vi "Lab Panel V4.83.vi"() -> ()   [LabVIEW 2013] (continued)
                            n2032 = Bundle By Name("Y"=w3252, "t0"=w3245) -> (w3244:waveform(dbl))  [unwired: 1 in]
                            n2033 = Bundle By Name("Y"=w3251, "t0"=w3245) -> (w3243:waveform(dbl))  [unwired: 1 in]
                            n2034 = Bundle By Name("Y"=w3250, "t0"=w3245) -> (w3242:waveform(dbl))  [unwired: 1 in]
                            n2035 = Bundle By Name("Y"=w3249, "t0"=w3245) -> (w3241:waveform(dbl))  [unwired: 1 in]
                            n2036 = Bundle By Name("Y"=w3248, "t0"=w3245) -> (w3240:waveform(dbl))  [unwired: 1 in]
                            n2037 = Bundle By Name("Y"=w3247, "t0"=w3245) -> (w3239:waveform(dbl))  [unwired: 1 in]
                            n2038 = Bundle By Name("Y"=w3246, "t0"=w3245) -> (w3238:waveform(dbl))  [unwired: 1 in]
                            n2039 = Build Array(w3244, w3243, w3242, w3241, w3240, w3239, w3238) -> (w3237:waveform(dbl)[])
                            n2040 = TDMS Write(0:w3258, 5:"TEST VALUES", 7:w3229, 9:w3237) -> (4:w3228:refnum<k34>, 6:w3227:string, 15:w3226:errorcluster)  [unwired: 2 in, 1 out]
                            n2041 = TDMS Write(0:w3228, 5:w3227, 7:"TIME", 9:w3224, 11:w3226) -> (15:w3223:errorcluster)  [unwired: 1 in, 3 out]
                            n2042 = local write "data file error"(w3223) -> ()
                          }
                        }
                      }
                    }
                  }
                }
              }
              frame #4 {
                n2043 = case shown="True" w3262 {
                  tunnel: w3266 -> [_ w3271]
                  tunnel: w3265 -> [_ w3270]
                  tunnel: w3264 -> [_ w3268]
                  tunnel: w3263 -> [_ w3267]
                  frame False {
                  }
                  frame True {
                    n2044 = local read "DISP LAB03-1"() -> (w3272:T4)
                    n2045 = local read "SIG LAB03-1"() -> (w3273:T2)
                    n2046 = local read "ON L03-1"() -> (w3269:cluster{"amps":dbl, "volts":dbl, "pf":dbl})
                    n2047 = Unbundle(w3273) -> ("AMPS"=w3279:dbl, "VOLTS"=w3277:dbl, "PF"=w3276:dbl, "Tmp Live"=w3275:dbl, "Tmp Neut"=w3278:dbl)
                    n2048 = Unbundle(w3272) -> ("CYCLE"=w3274:dbl)  [unwired: 2 out]
                    n2049 = stacked-sequence {
                      tunnel: w3279 -> [w3283 w3302]
                      tunnel: w3278 -> [_ w3301]
                      tunnel: w3277 -> [w3282 w3300]
                      tunnel: w3276 -> [w3281 w3299]
                      tunnel: w3275 -> [_ w3298]
                      tunnel: w3274 -> [_ w3297]
                      tunnel: w3271 -> [_ w3296]
                      tunnel: w3270 -> [w3284 _]
                      tunnel: w3269 -> [w3280 w3294]
                      tunnel: w3268 -> [_ w3295]
                      tunnel: w3267 -> [_ w3290]
                      frame #0 {
                        n2050 = case shown="True" w3284 {
                          tunnel: w3283 -> [_ w3289]
                          tunnel: w3282 -> [_ w3288]
                          tunnel: w3281 -> [_ w3287]
                          tunnel: w3280 -> [_ w3285]
                          frame False {
                          }
                          frame True {
                            n2051 = Bundle(cluster=w3285, "amps"=w3289, "volts"=w3288, "pf"=w3287) -> (w3286:cluster{"amps":dbl, "volts":dbl, "pf":dbl})
                            n2052 = local write "ON L03-1"(w3286) -> ()
                          }
                        }
                      }
                      frame #1 {
                        n2053 = Unbundle(w3294) -> ("amps"=w3293:dbl, "volts"=w3292:dbl, "pf"=w3291:dbl)
                        n2054 = case shown="True" w3295 {
                          tunnel: w3302 -> [_ w3334]
                          tunnel: w3301 -> [_ w3341]
                          tunnel: w3300 -> [_ _]
                          tunnel: w3299 -> [_ _]
                          tunnel: w3298 -> [_ w3340]
                          tunnel: w3297 -> [_ w3339]
                          tunnel: w3296 -> [_ w3304]
                          tunnel: w3293 -> [_ w3336]
                          tunnel: w3292 -> [_ w3335]
                          tunnel: w3291 -> [_ w3333]
                          tunnel: w3290 -> [_ w3325]
                          frame False {
                          }
                          frame True {
                            n2055 = local read "TDMS LAB03-1"() -> (w3338:refnum<k34>)
                            n2056 = Build Array(w3335) -> (w3330:dbl[])
                            n2057 = Build Array(w3333) -> (w3329:dbl[])
                            n2058 = Build Array(w3340) -> (w3328:dbl[])
                            n2059 = Build Array(w3341) -> (w3327:dbl[])
                            n2060 = Build Array(w3336) -> (w3332:dbl[])
                            n2061 = Build Array(w3334) -> (w3331:dbl[])
                            n2062 = Build Array(w3339) -> (w3326:dbl[])
                            n2063 = Build Array("AMPS ON", "AMPS OFF", "VOLTS", "PF", "TEMP Live", "TEMP Neut", "CYCLE") -> (w3309:string[])
                            n2064 = Bundle By Name("Y"=w3332, "t0"=w3325) -> (w3324:waveform(dbl))  [unwired: 1 in]
                            n2065 = Bundle By Name("Y"=w3331, "t0"=w3325) -> (w3323:waveform(dbl))  [unwired: 1 in]
                            n2066 = Bundle By Name("Y"=w3330, "t0"=w3325) -> (w3322:waveform(dbl))  [unwired: 1 in]
                            n2067 = Bundle By Name("Y"=w3329, "t0"=w3325) -> (w3321:waveform(dbl))  [unwired: 1 in]
                            n2068 = Bundle By Name("Y"=w3328, "t0"=w3325) -> (w3320:waveform(dbl))  [unwired: 1 in]
                            n2069 = Bundle By Name("Y"=w3327, "t0"=w3325) -> (w3319:waveform(dbl))  [unwired: 1 in]
                            n2070 = Bundle By Name("Y"=w3326, "t0"=w3325) -> (w3318:waveform(dbl))  [unwired: 1 in]
                            n2071 = Build Array(w3324, w3323, w3322, w3321, w3320, w3319, w3318) -> (w3317:waveform(dbl)[])
                            n2072 = TDMS Write(0:w3338, 5:"TEST VALUES", 7:w3309, 9:w3317) -> (4:w3308:refnum<k34>, 6:w3307:string, 15:w3306:errorcluster)  [unwired: 2 in, 1 out]
                            n2073 = TDMS Write(0:w3308, 5:w3307, 7:"TIME", 9:w3304, 11:w3306) -> (15:w3303:errorcluster)  [unwired: 1 in, 3 out]
                            n2074 = local write "data file error"(w3303) -> ()
                          }
                        }
                      }
                    }
                  }
                }
              }
              frame #5 {
                n2075 = case shown="True" w3342 {
                  tunnel: w3346 -> [_ w3351]
                  tunnel: w3345 -> [_ w3350]
                  tunnel: w3344 -> [_ w3348]
                  tunnel: w3343 -> [_ w3347]
                  frame False {
                  }
                  frame True {
                    n2076 = local read "DISP LAB03-2"() -> (w3352:T4)
                    n2077 = local read "SIG LAB03-2"() -> (w3353:T2)
                    n2078 = local read "ON L03-2"() -> (w3349:cluster{"amps":dbl, "volts":dbl, "pf":dbl})
                    n2079 = Unbundle(w3353) -> ("AMPS"=w3359:dbl, "VOLTS"=w3357:dbl, "PF"=w3356:dbl, "Tmp Live"=w3355:dbl, "Tmp Neut"=w3358:dbl)
                    n2080 = Unbundle(w3352) -> ("CYCLE"=w3354:dbl)  [unwired: 2 out]
                    n2081 = stacked-sequence {
                      tunnel: w3359 -> [w3363 w3382]
                      tunnel: w3358 -> [_ w3381]
                      tunnel: w3357 -> [w3362 w3380]
                      tunnel: w3356 -> [w3361 w3379]
                      tunnel: w3355 -> [_ w3378]
                      tunnel: w3354 -> [_ w3377]
                      tunnel: w3351 -> [_ w3376]
                      tunnel: w3350 -> [w3364 _]
                      tunnel: w3349 -> [w3360 w3374]
                      tunnel: w3348 -> [_ w3375]
                      tunnel: w3347 -> [_ w3370]
                      frame #0 {
                        n2082 = case shown="True" w3364 {
                          tunnel: w3363 -> [_ w3369]
                          tunnel: w3362 -> [_ w3368]
                          tunnel: w3361 -> [_ w3367]
                          tunnel: w3360 -> [_ w3365]
                          frame False {
                          }
                          frame True {
                            n2083 = Bundle(cluster=w3365, "amps"=w3369, "volts"=w3368, "pf"=w3367) -> (w3366:cluster{"amps":dbl, "volts":dbl, "pf":dbl})
                            n2084 = local write "ON L03-2"(w3366) -> ()
                          }
                        }
                      }
                      frame #1 {
                        n2085 = Unbundle(w3374) -> ("amps"=w3373:dbl, "volts"=w3372:dbl, "pf"=w3371:dbl)
                        n2086 = case shown="True" w3375 {
                          tunnel: w3382 -> [_ w3414]
                          tunnel: w3381 -> [_ w3421]
                          tunnel: w3380 -> [_ _]
                          tunnel: w3379 -> [_ _]
                          tunnel: w3378 -> [_ w3420]
                          tunnel: w3377 -> [_ w3419]
                          tunnel: w3376 -> [_ w3384]
                          tunnel: w3373 -> [_ w3416]
                          tunnel: w3372 -> [_ w3415]
                          tunnel: w3371 -> [_ w3413]
                          tunnel: w3370 -> [_ w3405]
                          frame False {
                          }
                          frame True {
                            n2087 = local read "TDMS LAB03-2"() -> (w3418:refnum<k34>)
                            n2088 = Build Array(w3415) -> (w3410:dbl[])
                            n2089 = Build Array(w3413) -> (w3409:dbl[])
                            n2090 = Build Array(w3420) -> (w3408:dbl[])
                            n2091 = Build Array(w3421) -> (w3407:dbl[])
                            n2092 = Build Array(w3416) -> (w3412:dbl[])
                            n2093 = Build Array(w3414) -> (w3411:dbl[])
                            n2094 = Build Array(w3419) -> (w3406:dbl[])
                            n2095 = Build Array("AMPS ON", "AMPS OFF", "VOLTS", "PF", "TEMP Live", "TEMP Neut", "CYCLE") -> (w3389:string[])
                            n2096 = Bundle By Name("Y"=w3412, "t0"=w3405) -> (w3404:waveform(dbl))  [unwired: 1 in]
                            n2097 = Bundle By Name("Y"=w3411, "t0"=w3405) -> (w3403:waveform(dbl))  [unwired: 1 in]
                            n2098 = Bundle By Name("Y"=w3410, "t0"=w3405) -> (w3402:waveform(dbl))  [unwired: 1 in]
                            n2099 = Bundle By Name("Y"=w3409, "t0"=w3405) -> (w3401:waveform(dbl))  [unwired: 1 in]
                            n2100 = Bundle By Name("Y"=w3408, "t0"=w3405) -> (w3400:waveform(dbl))  [unwired: 1 in]
                            n2101 = Bundle By Name("Y"=w3407, "t0"=w3405) -> (w3399:waveform(dbl))  [unwired: 1 in]
                            n2102 = Bundle By Name("Y"=w3406, "t0"=w3405) -> (w3398:waveform(dbl))  [unwired: 1 in]
                            n2103 = Build Array(w3404, w3403, w3402, w3401, w3400, w3399, w3398) -> (w3397:waveform(dbl)[])
                            n2104 = TDMS Write(0:w3418, 5:"TEST VALUES", 7:w3389, 9:w3397) -> (4:w3388:refnum<k34>, 6:w3387:string, 15:w3386:errorcluster)  [unwired: 2 in, 1 out]
                            n2105 = TDMS Write(0:w3388, 5:w3387, 7:"TIME", 9:w3384, 11:w3386) -> (15:w3383:errorcluster)  [unwired: 1 in, 3 out]
                            n2106 = local write "data file error"(w3383) -> ()
                          }
                        }
                      }
                    }
                  }
                }
              }
              frame #6 {
                n2107 = case shown="True" w3422 {
                  tunnel: w3426 -> [_ w3431]
                  tunnel: w3425 -> [_ w3430]
                  tunnel: w3424 -> [_ w3428]
                  tunnel: w3423 -> [_ w3427]
                  frame False {
                  }
                  frame True {
                    n2108 = local read "DISP LAB04-1"() -> (w3432:T4)
                    n2109 = local read "SIG LAB04-1"() -> (w3433:T2)
                    n2110 = local read "ON L04-1"() -> (w3429:cluster{"amps":dbl, "volts":dbl, "pf":dbl})
                    n2111 = Unbundle(w3433) -> ("AMPS"=w3439:dbl, "VOLTS"=w3437:dbl, "PF"=w3436:dbl, "Tmp Live"=w3435:dbl, "Tmp Neut"=w3438:dbl)
                    n2112 = Unbundle(w3432) -> ("CYCLE"=w3434:dbl)  [unwired: 2 out]
                    n2113 = stacked-sequence {
                      tunnel: w3439 -> [w3443 w3462]
                      tunnel: w3438 -> [_ w3461]
                      tunnel: w3437 -> [w3442 w3460]
                      tunnel: w3436 -> [w3441 w3459]
                      tunnel: w3435 -> [_ w3458]
                      tunnel: w3434 -> [_ w3457]
                      tunnel: w3431 -> [_ w3456]
                      tunnel: w3430 -> [w3444 _]
                      tunnel: w3429 -> [w3440 w3454]
                      tunnel: w3428 -> [_ w3455]
                      tunnel: w3427 -> [_ w3450]
                      frame #0 {
                        n2114 = case shown="True" w3444 {
                          tunnel: w3443 -> [_ w3449]
                          tunnel: w3442 -> [_ w3448]
                          tunnel: w3441 -> [_ w3447]
                          tunnel: w3440 -> [_ w3445]
                          frame False {
                          }
                          frame True {
                            n2115 = Bundle(cluster=w3445, "amps"=w3449, "volts"=w3448, "pf"=w3447) -> (w3446:cluster{"amps":dbl, "volts":dbl, "pf":dbl})
                            n2116 = local write "ON L04-1"(w3446) -> ()
                          }
                        }
                      }
                      frame #1 {
                        n2117 = Unbundle(w3454) -> ("amps"=w3453:dbl, "volts"=w3452:dbl, "pf"=w3451:dbl)
                        n2118 = case shown="True" w3455 {
                          tunnel: w3462 -> [_ w3494]
                          tunnel: w3461 -> [_ w3501]
                          tunnel: w3460 -> [_ _]
                          tunnel: w3459 -> [_ _]
                          tunnel: w3458 -> [_ w3500]
                          tunnel: w3457 -> [_ w3499]
                          tunnel: w3456 -> [_ w3464]
                          tunnel: w3453 -> [_ w3496]
                          tunnel: w3452 -> [_ w3495]
                          tunnel: w3451 -> [_ w3493]
                          tunnel: w3450 -> [_ w3485]
                          frame False {
                          }
                          frame True {
                            n2119 = local read "TDMS LAB04-1"() -> (w3498:refnum<k34>)
                            n2120 = Build Array(w3495) -> (w3490:dbl[])
                            n2121 = Build Array(w3493) -> (w3489:dbl[])
                            n2122 = Build Array(w3500) -> (w3488:dbl[])
                            n2123 = Build Array(w3501) -> (w3487:dbl[])
                            n2124 = Build Array(w3496) -> (w3492:dbl[])
                            n2125 = Build Array(w3494) -> (w3491:dbl[])
                            n2126 = Build Array(w3499) -> (w3486:dbl[])
                            n2127 = Build Array("AMPS ON", "AMPS OFF", "VOLTS", "PF", "TEMP Live", "TEMP Neut", "CYCLE") -> (w3469:string[])
                            n2128 = Bundle By Name("Y"=w3492, "t0"=w3485) -> (w3484:waveform(dbl))  [unwired: 1 in]
                            n2129 = Bundle By Name("Y"=w3491, "t0"=w3485) -> (w3483:waveform(dbl))  [unwired: 1 in]
                            n2130 = Bundle By Name("Y"=w3490, "t0"=w3485) -> (w3482:waveform(dbl))  [unwired: 1 in]
                            n2131 = Bundle By Name("Y"=w3489, "t0"=w3485) -> (w3481:waveform(dbl))  [unwired: 1 in]
                            n2132 = Bundle By Name("Y"=w3488, "t0"=w3485) -> (w3480:waveform(dbl))  [unwired: 1 in]
                            n2133 = Bundle By Name("Y"=w3487, "t0"=w3485) -> (w3479:waveform(dbl))  [unwired: 1 in]
                            n2134 = Bundle By Name("Y"=w3486, "t0"=w3485) -> (w3478:waveform(dbl))  [unwired: 1 in]
                            n2135 = Build Array(w3484, w3483, w3482, w3481, w3480, w3479, w3478) -> (w3477:waveform(dbl)[])
                            n2136 = TDMS Write(0:w3498, 5:"TEST VALUES", 7:w3469, 9:w3477) -> (4:w3468:refnum<k34>, 6:w3467:string, 15:w3466:errorcluster)  [unwired: 2 in, 1 out]
                            n2137 = TDMS Write(0:w3468, 5:w3467, 7:"TIME", 9:w3464, 11:w3466) -> (15:w3463:errorcluster)  [unwired: 1 in, 3 out]
                            n2138 = local write "data file error"(w3463) -> ()
                          }
                        }
                      }
                    }
                  }
                }
              }
              frame #7 {
                n2139 = case shown="True" w3502 {
                  tunnel: w3506 -> [_ w3511]
                  tunnel: w3505 -> [_ w3510]
                  tunnel: w3504 -> [_ w3508]
                  tunnel: w3503 -> [_ w3507]
                  frame False {
                  }
                  frame True {
                    n2140 = local read "DISP LAB04-2"() -> (w3512:T4)
                    n2141 = local read "SIG LAB04-2"() -> (w3513:T2)
                    n2142 = local read "ON L04-2"() -> (w3509:cluster{"amps":dbl, "volts":dbl, "pf":dbl})
                    n2143 = Unbundle(w3513) -> ("AMPS"=w3519:dbl, "VOLTS"=w3517:dbl, "PF"=w3516:dbl, "Tmp Live"=w3515:dbl, "Tmp Neut"=w3518:dbl)
                    n2144 = Unbundle(w3512) -> ("CYCLE"=w3514:dbl)  [unwired: 2 out]
                    n2145 = stacked-sequence {
                      tunnel: w3519 -> [w3523 w3542]
                      tunnel: w3518 -> [_ w3541]
                      tunnel: w3517 -> [w3522 w3540]
                      tunnel: w3516 -> [w3521 w3539]
                      tunnel: w3515 -> [_ w3538]
                      tunnel: w3514 -> [_ w3537]
                      tunnel: w3511 -> [_ w3536]
                      tunnel: w3510 -> [w3524 _]
                      tunnel: w3509 -> [w3520 w3534]
                      tunnel: w3508 -> [_ w3535]
                      tunnel: w3507 -> [_ w3530]
                      frame #0 {
                        n2146 = case shown="True" w3524 {
                          tunnel: w3523 -> [_ w3529]
                          tunnel: w3522 -> [_ w3528]
                          tunnel: w3521 -> [_ w3527]
                          tunnel: w3520 -> [_ w3525]
                          frame False {
                          }
                          frame True {
                            n2147 = Bundle(cluster=w3525, "amps"=w3529, "volts"=w3528, "pf"=w3527) -> (w3526:cluster{"amps":dbl, "volts":dbl, "pf":dbl})
                            n2148 = local write "ON L04-2"(w3526) -> ()
                          }
                        }
                      }
                      frame #1 {
                        n2149 = Unbundle(w3534) -> ("amps"=w3533:dbl, "volts"=w3532:dbl, "pf"=w3531:dbl)
                        n2150 = case shown="True" w3535 {
                          tunnel: w3542 -> [_ w3574]
                          tunnel: w3541 -> [_ w3581]
                          tunnel: w3540 -> [_ _]
                          tunnel: w3539 -> [_ _]
                          tunnel: w3538 -> [_ w3580]
                          tunnel: w3537 -> [_ w3579]
                          tunnel: w3536 -> [_ w3544]
                          tunnel: w3533 -> [_ w3576]
                          tunnel: w3532 -> [_ w3575]
                          tunnel: w3531 -> [_ w3573]
                          tunnel: w3530 -> [_ w3565]
                          frame False {
                          }
                          frame True {
                            n2151 = local read "TDMS LAB04-2"() -> (w3578:refnum<k34>)
                            n2152 = Build Array(w3575) -> (w3570:dbl[])
                            n2153 = Build Array(w3573) -> (w3569:dbl[])
                            n2154 = Build Array(w3580) -> (w3568:dbl[])
                            n2155 = Build Array(w3581) -> (w3567:dbl[])
                            n2156 = Build Array(w3576) -> (w3572:dbl[])
                            n2157 = Build Array(w3574) -> (w3571:dbl[])
                            n2158 = Build Array(w3579) -> (w3566:dbl[])
                            n2159 = Build Array("AMPS ON", "AMPS OFF", "VOLTS", "PF", "TEMP Live", "TEMP Neut", "CYCLE") -> (w3549:string[])
                            n2160 = Bundle By Name("Y"=w3572, "t0"=w3565) -> (w3564:waveform(dbl))  [unwired: 1 in]
                            n2161 = Bundle By Name("Y"=w3571, "t0"=w3565) -> (w3563:waveform(dbl))  [unwired: 1 in]
                            n2162 = Bundle By Name("Y"=w3570, "t0"=w3565) -> (w3562:waveform(dbl))  [unwired: 1 in]
                            n2163 = Bundle By Name("Y"=w3569, "t0"=w3565) -> (w3561:waveform(dbl))  [unwired: 1 in]
                            n2164 = Bundle By Name("Y"=w3568, "t0"=w3565) -> (w3560:waveform(dbl))  [unwired: 1 in]
                            n2165 = Bundle By Name("Y"=w3567, "t0"=w3565) -> (w3559:waveform(dbl))  [unwired: 1 in]
                            n2166 = Bundle By Name("Y"=w3566, "t0"=w3565) -> (w3558:waveform(dbl))  [unwired: 1 in]
                            n2167 = Build Array(w3564, w3563, w3562, w3561, w3560, w3559, w3558) -> (w3557:waveform(dbl)[])
                            n2168 = TDMS Write(0:w3578, 5:"TEST VALUES", 7:w3549, 9:w3557) -> (4:w3548:refnum<k34>, 6:w3547:string, 15:w3546:errorcluster)  [unwired: 2 in, 1 out]
                            n2169 = TDMS Write(0:w3548, 5:w3547, 7:"TIME", 9:w3544, 11:w3546) -> (15:w3543:errorcluster)  [unwired: 1 in, 3 out]
                            n2170 = local write "data file error"(w3543) -> ()
                          }
                        }
                      }
                    }
                  }
                }
              }
              frame #8 {
                n2171 = case shown="True" w3582 {
                  tunnel: w3586 -> [_ w3591]
                  tunnel: w3585 -> [_ w3590]
                  tunnel: w3584 -> [_ w3588]
                  tunnel: w3583 -> [_ w3587]
                  frame False {
                  }
                  frame True {
                    n2172 = local read "DISP LAB05-1"() -> (w3592:T4)
                    n2173 = local read "SIG LAB05-1"() -> (w3593:T2)
                    n2174 = local read "ON L05-1"() -> (w3589:cluster{"amps":dbl, "volts":dbl, "pf":dbl})
                    n2175 = Unbundle(w3593) -> ("AMPS"=w3599:dbl, "VOLTS"=w3597:dbl, "PF"=w3596:dbl, "Tmp Live"=w3595:dbl, "Tmp Neut"=w3598:dbl)
                    n2176 = Unbundle(w3592) -> ("CYCLE"=w3594:dbl)  [unwired: 2 out]
                    n2177 = stacked-sequence {
                      tunnel: w3599 -> [w3603 w3622]
                      tunnel: w3598 -> [_ w3621]
                      tunnel: w3597 -> [w3602 w3620]
                      tunnel: w3596 -> [w3601 w3619]
                      tunnel: w3595 -> [_ w3618]
                      tunnel: w3594 -> [_ w3617]
                      tunnel: w3591 -> [_ w3616]
                      tunnel: w3590 -> [w3604 _]
                      tunnel: w3589 -> [w3600 w3614]
                      tunnel: w3588 -> [_ w3615]
                      tunnel: w3587 -> [_ w3610]
                      frame #0 {
                        n2178 = case shown="True" w3604 {
                          tunnel: w3603 -> [_ w3609]
                          tunnel: w3602 -> [_ w3608]
                          tunnel: w3601 -> [_ w3607]
                          tunnel: w3600 -> [_ w3605]
                          frame False {
                          }
                          frame True {
                            n2179 = Bundle(cluster=w3605, "amps"=w3609, "volts"=w3608, "pf"=w3607) -> (w3606:cluster{"amps":dbl, "volts":dbl, "pf":dbl})
                            n2180 = local write "ON L05-1"(w3606) -> ()
                          }
                        }
                      }
                      frame #1 {
                        n2181 = Unbundle(w3614) -> ("amps"=w3613:dbl, "volts"=w3612:dbl, "pf"=w3611:dbl)
                        n2182 = case shown="True" w3615 {
                          tunnel: w3622 -> [_ w3654]
                          tunnel: w3621 -> [_ w3661]
                          tunnel: w3620 -> [_ _]
                          tunnel: w3619 -> [_ _]
                          tunnel: w3618 -> [_ w3660]
                          tunnel: w3617 -> [_ w3659]
                          tunnel: w3616 -> [_ w3624]
                          tunnel: w3613 -> [_ w3656]
                          tunnel: w3612 -> [_ w3655]
                          tunnel: w3611 -> [_ w3653]
                          tunnel: w3610 -> [_ w3645]
                          frame False {
                          }
                          frame True {
                            n2183 = local read "TDMS LAB05-1"() -> (w3658:refnum<k34>)
                            n2184 = Build Array(w3655) -> (w3650:dbl[])
                            n2185 = Build Array(w3653) -> (w3649:dbl[])
                            n2186 = Build Array(w3660) -> (w3648:dbl[])
                            n2187 = Build Array(w3661) -> (w3647:dbl[])
                            n2188 = Build Array(w3656) -> (w3652:dbl[])
                            n2189 = Build Array(w3654) -> (w3651:dbl[])
                            n2190 = Build Array(w3659) -> (w3646:dbl[])
                            n2191 = Build Array("AMPS ON", "AMPS OFF", "VOLTS", "PF", "TEMP Live", "TEMP Neut", "CYCLE") -> (w3629:string[])
                            n2192 = Bundle By Name("Y"=w3652, "t0"=w3645) -> (w3644:waveform(dbl))  [unwired: 1 in]
                            n2193 = Bundle By Name("Y"=w3651, "t0"=w3645) -> (w3643:waveform(dbl))  [unwired: 1 in]
                            n2194 = Bundle By Name("Y"=w3650, "t0"=w3645) -> (w3642:waveform(dbl))  [unwired: 1 in]
                            n2195 = Bundle By Name("Y"=w3649, "t0"=w3645) -> (w3641:waveform(dbl))  [unwired: 1 in]
                            n2196 = Bundle By Name("Y"=w3648, "t0"=w3645) -> (w3640:waveform(dbl))  [unwired: 1 in]
                            n2197 = Bundle By Name("Y"=w3647, "t0"=w3645) -> (w3639:waveform(dbl))  [unwired: 1 in]
                            n2198 = Bundle By Name("Y"=w3646, "t0"=w3645) -> (w3638:waveform(dbl))  [unwired: 1 in]
                            n2199 = Build Array(w3644, w3643, w3642, w3641, w3640, w3639, w3638) -> (w3637:waveform(dbl)[])
                            n2200 = TDMS Write(0:w3658, 5:"TEST VALUES", 7:w3629, 9:w3637) -> (4:w3628:refnum<k34>, 6:w3627:string, 15:w3626:errorcluster)  [unwired: 2 in, 1 out]
                            n2201 = TDMS Write(0:w3628, 5:w3627, 7:"TIME", 9:w3624, 11:w3626) -> (15:w3623:errorcluster)  [unwired: 1 in, 3 out]
                            n2202 = local write "data file error"(w3623) -> ()
                          }
                        }
                      }
                    }
                  }
                }
              }
              frame #9 {
                n2203 = case shown="True" w3662 {
                  tunnel: w3666 -> [_ w3671]
                  tunnel: w3665 -> [_ w3670]
                  tunnel: w3664 -> [_ w3668]
                  tunnel: w3663 -> [_ w3667]
                  frame False {
                  }
                  frame True {
                    n2204 = local read "DISP LAB05-2"() -> (w3672:T4)
                    n2205 = local read "SIG LAB05-2"() -> (w3673:T2)
                    n2206 = local read "ON L05-2"() -> (w3669:cluster{"amps":dbl, "volts":dbl, "pf":dbl})
                    n2207 = Unbundle(w3673) -> ("AMPS"=w3679:dbl, "VOLTS"=w3677:dbl, "PF"=w3676:dbl, "Tmp Live"=w3675:dbl, "Tmp Neut"=w3678:dbl)
                    n2208 = Unbundle(w3672) -> ("CYCLE"=w3674:dbl)  [unwired: 2 out]
                    n2209 = stacked-sequence {
                      tunnel: w3679 -> [w3683 w3702]
                      tunnel: w3678 -> [_ w3701]
                      tunnel: w3677 -> [w3682 w3700]
                      tunnel: w3676 -> [w3681 w3699]
                      tunnel: w3675 -> [_ w3698]
                      tunnel: w3674 -> [_ w3697]
                      tunnel: w3671 -> [_ w3696]
                      tunnel: w3670 -> [w3684 _]
                      tunnel: w3669 -> [w3680 w3694]
                      tunnel: w3668 -> [_ w3695]
                      tunnel: w3667 -> [_ w3690]
                      frame #0 {
                        n2210 = case shown="True" w3684 {
                          tunnel: w3683 -> [_ w3689]
                          tunnel: w3682 -> [_ w3688]
                          tunnel: w3681 -> [_ w3687]
                          tunnel: w3680 -> [_ w3685]
                          frame False {
                          }
                          frame True {
                            n2211 = Bundle(cluster=w3685, "amps"=w3689, "volts"=w3688, "pf"=w3687) -> (w3686:cluster{"amps":dbl, "volts":dbl, "pf":dbl})
                            n2212 = local write "ON L05-2"(w3686) -> ()
                          }
                        }
                      }
                      frame #1 {
                        n2213 = Unbundle(w3694) -> ("amps"=w3693:dbl, "volts"=w3692:dbl, "pf"=w3691:dbl)
                        n2214 = case shown="True" w3695 {
                          tunnel: w3702 -> [_ w3734]
                          tunnel: w3701 -> [_ w3741]
                          tunnel: w3700 -> [_ _]
                          tunnel: w3699 -> [_ _]
                          tunnel: w3698 -> [_ w3740]
                          tunnel: w3697 -> [_ w3739]
                          tunnel: w3696 -> [_ w3704]
                          tunnel: w3693 -> [_ w3736]
                          tunnel: w3692 -> [_ w3735]
                          tunnel: w3691 -> [_ w3733]
                          tunnel: w3690 -> [_ w3725]
                          frame False {
                          }
                          frame True {
                            n2215 = local read "TDMS LAB05-2"() -> (w3738:refnum<k34>)
                            n2216 = Build Array(w3735) -> (w3730:dbl[])
                            n2217 = Build Array(w3733) -> (w3729:dbl[])
                            n2218 = Build Array(w3740) -> (w3728:dbl[])
                            n2219 = Build Array(w3741) -> (w3727:dbl[])
                            n2220 = Build Array(w3736) -> (w3732:dbl[])
                            n2221 = Build Array(w3734) -> (w3731:dbl[])
                            n2222 = Build Array(w3739) -> (w3726:dbl[])
                            n2223 = Build Array("AMPS ON", "AMPS OFF", "VOLTS", "PF", "TEMP Live", "TEMP Neut", "CYCLE") -> (w3709:string[])
                            n2224 = Bundle By Name("Y"=w3732, "t0"=w3725) -> (w3724:waveform(dbl))  [unwired: 1 in]
                            n2225 = Bundle By Name("Y"=w3731, "t0"=w3725) -> (w3723:waveform(dbl))  [unwired: 1 in]
                            n2226 = Bundle By Name("Y"=w3730, "t0"=w3725) -> (w3722:waveform(dbl))  [unwired: 1 in]
                            n2227 = Bundle By Name("Y"=w3729, "t0"=w3725) -> (w3721:waveform(dbl))  [unwired: 1 in]
                            n2228 = Bundle By Name("Y"=w3728, "t0"=w3725) -> (w3720:waveform(dbl))  [unwired: 1 in]
                            n2229 = Bundle By Name("Y"=w3727, "t0"=w3725) -> (w3719:waveform(dbl))  [unwired: 1 in]
                            n2230 = Bundle By Name("Y"=w3726, "t0"=w3725) -> (w3718:waveform(dbl))  [unwired: 1 in]
                            n2231 = Build Array(w3724, w3723, w3722, w3721, w3720, w3719, w3718) -> (w3717:waveform(dbl)[])
                            n2232 = TDMS Write(0:w3738, 5:"TEST VALUES", 7:w3709, 9:w3717) -> (4:w3708:refnum<k34>, 6:w3707:string, 15:w3706:errorcluster)  [unwired: 2 in, 1 out]
                            n2233 = TDMS Write(0:w3708, 5:w3707, 7:"TIME", 9:w3704, 11:w3706) -> (15:w3703:errorcluster)  [unwired: 1 in, 3 out]
                            n2234 = local write "data file error"(w3703) -> ()
                          }
                        }
                      }
                    }
                  }
                }
              }
            }
          }
          frame #13 {
            # "display test values on chart"
            n2235 = case shown="\"OFF CYCLE\"" "Select  Cycle" {
              tunnel: [1 w3747] -> w3742
              frame "ON CYCLE", Default {
              }
              frame "OFF CYCLE" {
                n2236 = local read "on loops"() -> (w3749:dbl)
                n2237 = Add(x=w3749, y=2) -> (x+y=w3747:dbl)
              }
            }
            n2238 = local read "jig cycle"() -> (w3744:dbl)
            n2239 = Equal?(x=w3744, y=w3742) -> (x = y?=w3745:bool)
            n2240 = case shown="True" w3745 {
              frame False {
              }
              frame True {
                n2241 = local read "SIG LAB05-1"() -> (w3791:T2)
                n2242 = local read "SIG LAB04-2"() -> (w3792:T2)
                n2243 = local read "SIG LAB05-2"() -> (w3790:T2)
                n2244 = local read "SIG LAB04-1"() -> (w3793:T2)
                n2245 = local read "SIG LAB03-1"() -> (w3795:T2)
                n2246 = local read "SIG LAB03-2"() -> (w3794:T2)
                n2247 = local read "SIG LAB01-1"() -> (w3799:T2)
                n2248 = local read "SIG LAB02-2"() -> (w3796:T2)
                n2249 = local read "SIG LAB02-1"() -> (w3797:T2)
                n2250 = local read "SIG LAB01-2"() -> (w3798:T2)
                n2251 = Unbundle(w3792) -> ("AMPS"=w3782:dbl, "VOLTS"=w3772:dbl, "Tmp Live"=w3762:dbl, "Tmp Neut"=w3752:dbl)  [unwired: 1 out]
                n2252 = Unbundle(w3791) -> ("AMPS"=w3781:dbl, "VOLTS"=w3771:dbl, "Tmp Live"=w3761:dbl, "Tmp Neut"=w3751:dbl)  [unwired: 1 out]
                n2253 = Unbundle(w3790) -> ("AMPS"=w3780:dbl, "VOLTS"=w3770:dbl, "Tmp Live"=w3760:dbl, "Tmp Neut"=w3750:dbl)  [unwired: 1 out]
                n2254 = Unbundle(w3793) -> ("AMPS"=w3783:dbl, "VOLTS"=w3773:dbl, "Tmp Live"=w3763:dbl, "Tmp Neut"=w3753:dbl)  [unwired: 1 out]
                n2255 = Unbundle(w3794) -> ("AMPS"=w3784:dbl, "VOLTS"=w3774:dbl, "Tmp Live"=w3764:dbl, "Tmp Neut"=w3754:dbl)  [unwired: 1 out]
                n2256 = Unbundle(w3795) -> ("AMPS"=w3785:dbl, "VOLTS"=w3775:dbl, "Tmp Live"=w3765:dbl, "Tmp Neut"=w3755:dbl)  [unwired: 1 out]
                n2257 = Unbundle(w3796) -> ("AMPS"=w3786:dbl, "VOLTS"=w3776:dbl, "Tmp Live"=w3766:dbl, "Tmp Neut"=w3756:dbl)  [unwired: 1 out]
                n2258 = Unbundle(w3797) -> ("AMPS"=w3787:dbl, "VOLTS"=w3777:dbl, "Tmp Live"=w3767:dbl, "Tmp Neut"=w3757:dbl)  [unwired: 1 out]
                n2259 = Unbundle(w3799) -> ("AMPS"=w3789:dbl, "VOLTS"=w3779:dbl, "Tmp Live"=w3769:dbl, "Tmp Neut"=w3759:dbl)  [unwired: 1 out]
                n2260 = Unbundle(w3798) -> ("AMPS"=w3788:dbl, "VOLTS"=w3778:dbl, "Tmp Live"=w3768:dbl, "Tmp Neut"=w3758:dbl)  [unwired: 1 out]
                n2261 = stacked-sequence {
                  tunnel: w3789 -> [w3810 _ _ _]
                  tunnel: w3788 -> [w3809 _ _ _]
                  tunnel: w3787 -> [w3808 _ _ _]
                  tunnel: w3786 -> [w3807 _ _ _]
                  tunnel: w3785 -> [w3806 _ _ _]
                  tunnel: w3784 -> [w3805 _ _ _]
                  tunnel: w3783 -> [w3804 _ _ _]
                  tunnel: w3782 -> [w3803 _ _ _]
                  tunnel: w3781 -> [w3802 _ _ _]
                  tunnel: w3780 -> [w3801 _ _ _]
                  tunnel: w3779 -> [_ w3821 _ _]
                  tunnel: w3778 -> [_ w3820 _ _]
                  tunnel: w3777 -> [_ w3819 _ _]
                  tunnel: w3776 -> [_ w3818 _ _]
                  tunnel: w3775 -> [_ w3817 _ _]
                  tunnel: w3774 -> [_ w3816 _ _]
                  tunnel: w3773 -> [_ w3815 _ _]
                  tunnel: w3772 -> [_ w3814 _ _]
                  tunnel: w3771 -> [_ w3813 _ _]
                  tunnel: w3770 -> [_ w3812 _ _]
                  tunnel: w3769 -> [_ _ w3832 _]
                  tunnel: w3768 -> [_ _ w3831 _]
                  tunnel: w3767 -> [_ _ w3830 _]
                  tunnel: w3766 -> [_ _ w3829 _]
                  tunnel: w3765 -> [_ _ w3828 _]
                  tunnel: w3764 -> [_ _ w3827 _]
                  tunnel: w3763 -> [_ _ w3826 _]
                  tunnel: w3762 -> [_ _ w3825 _]
                  tunnel: w3761 -> [_ _ w3824 _]
                  tunnel: w3760 -> [_ _ w3823 _]
                  tunnel: w3759 -> [_ _ _ w3843]
                  tunnel: w3758 -> [_ _ _ w3842]
                  tunnel: w3757 -> [_ _ _ w3841]
                  tunnel: w3756 -> [_ _ _ w3840]
                  tunnel: w3755 -> [_ _ _ w3839]
                  tunnel: w3754 -> [_ _ _ w3838]
                  tunnel: w3753 -> [_ _ _ w3837]
                  tunnel: w3752 -> [_ _ _ w3836]
                  tunnel: w3751 -> [_ _ _ w3835]
                  tunnel: w3750 -> [_ _ _ w3834]
                  frame #0 {
                    n2262 = Merge Signals(w3810, w3809, w3808, w3807, w3806, w3805, w3804, w3803, w3802, w3801) -> (w3800:dynamicdata)
                    "TEST AMPS CHART" <- w3800
                    n2263 = global write "Global display 3.vi" "TEST AMPS CHART"(w3800) -> ()
                  }
                  frame #1 {
                    n2264 = Merge Signals(w3821, w3820, w3819, w3818, w3817, w3816, w3815, w3814, w3813, w3812) -> (w3811:dynamicdata)
                    "TEST VOLTS CHART" <- w3811
                    n2265 = global write "Global display 3.vi" "TEST VOLTS CHART"(w3811) -> ()
                  }
                  frame #2 {
                    n2266 = Merge Signals(w3832, w3831, w3830, w3829, w3828, w3827, w3826, w3825, w3824, w3823) -> (w3822:dynamicdata)
                    "TEMPERATURE (L) CHART" <- w3822
                    n2267 = global write "Global display 3.vi" "TEMPERATURE (L) CHART"(w3822) -> ()
                  }
                  frame #3 {
                    n2268 = Merge Signals(w3843, w3842, w3841, w3840, w3839, w3838, w3837, w3836, w3835, w3834) -> (w3833:dynamicdata)
                    "TEMPERATURE (N) CHART" <- w3833
                    n2269 = global write "Global display 3.vi" "TEMPERATURE (N) CHART"(w3833) -> ()
                  }
                }
              }
            }
          }
          frame #14 {
            # "check for amps fail"
            # "check for cycle test & temperature rise fail conditions"
            n2270 = local read "on loops"() -> (w3870:dbl)
            n2271 = local read "jig cycle"() -> (w3867:dbl)
            n2272 = local read "jig cycle"() -> (w3872:dbl)
            n2273 = Add(x=w3870, y=3.0) -> (x+y=w3868:dbl)
            n2274 = Equal?(x=w3867, y=w3868) -> (x = y?=w3863:bool)
            n2275 = local read "Fail Loops"() -> (w3844:dbl)
            n2276 = Equal?(x=w3872, y=1.0) -> (x = y?=w3865:bool)
            n2277 = global write "Global 1.vi" "fail count"(w3844) -> ()
            n2278 = stacked-sequence {
              tunnel: w3866 -> [w3875 _ _ _ _ _ _ _ _ _]
              tunnel: w3865 -> [w3876 w3896 w3916 w3936 w3956 w3976 w3996 w4016 w4036 w4056]
              tunnel: w3864 -> [w3873 _ _ _ _ _ _ _ _ _]
              tunnel: w3863 -> [w3874 w3895 w3915 w3935 w3955 w3975 w3995 w4015 w4035 w4055]
              tunnel: w3862 -> [_ w3894 _ _ _ _ _ _ _ _]
              tunnel: w3861 -> [_ w3893 _ _ _ _ _ _ _ _]
              tunnel: w3860 -> [_ _ w3914 _ _ _ _ _ _ _]
              tunnel: w3859 -> [_ _ w3913 _ _ _ _ _ _ _]
              tunnel: w3858 -> [_ _ _ w3934 _ _ _ _ _ _]
              tunnel: w3857 -> [_ _ _ w3933 _ _ _ _ _ _]
              tunnel: w3856 -> [_ _ _ _ w3954 _ _ _ _ _]
              tunnel: w3855 -> [_ _ _ _ w3953 _ _ _ _ _]
              tunnel: w3854 -> [_ _ _ _ _ w3974 _ _ _ _]
              tunnel: w3853 -> [_ _ _ _ _ w3973 _ _ _ _]
              tunnel: w3852 -> [_ _ _ _ _ _ w3994 _ _ _]
              tunnel: w3851 -> [_ _ _ _ _ _ w3993 _ _ _]
              tunnel: w3850 -> [_ _ _ _ _ _ _ w4014 _ _]
              tunnel: w3849 -> [_ _ _ _ _ _ _ w4013 _ _]
              tunnel: w3848 -> [_ _ _ _ _ _ _ _ w4034 _]
              tunnel: w3847 -> [_ _ _ _ _ _ _ _ w4033 _]
              tunnel: w3846 -> [_ _ _ _ _ _ _ _ _ w4054]
              tunnel: w3845 -> [_ _ _ _ _ _ _ _ _ w4053]
              frame #0 {
                # "LAB01-1"
                n2279 = case shown="True" w3873 {
                  tunnel: w3876 -> [_ w3889]
                  tunnel: w3875 -> [_ w3886]
                  tunnel: w3874 -> [_ w3885]
                  frame False {
                  }
                  frame True {
                    n2280 = local read "TEMP START LAB01-1"() -> (w3891:cluster{"TL":dbl, "TN":dbl})
                    n2281 = local read "RESULT LAB01-1"() -> (w3880:bool)
                    n2282 = local read "FAIL LAB01-1"() -> (w3883:cluster{"LO":dbl, "HI":dbl})
                    n2283 = local read "TDMS LAB01-1"() -> (w3890:refnum<k34>)
                    n2284 = local read "SET LAB01-1"() -> (w3887:T5)
                    n2285 = local read "DISP LAB01-1"() -> (w3888:T4)
                    n2286 = local read "SIG LAB01-1"() -> (w3892:T2)
                    n2287 = Bundle("FAIL LAB01-1"=w3883, "SIG LAB01-1"=w3892, "TEMP START LAB01-1"=w3891, "DISP LAB01-1"=w3888, "SET LAB01-1"=w3887, "TDMS LAB01-1"=w3890) -> (w3877:T28)  [unwired: 1 in]
                    n2288 = call "sub vi - cycle&temp fail v6.vi"("Amps Lo?"=w3889, "Input Cluster"=w3877, "SELECT"=w3886, "Amps Hi?"=w3885, "Result In"=w3880) -> ("(FAIL) out"=w3882:cluster{"FAIL LO":dbl, "FAIL HI":dbl}, "(DISP) out"=w3878:T4, "T-RISE"=w3879:cluster{"T-RISE (L)":dbl, "T-RISE (N)":dbl}, "Result Out"=w3881:bool, "file error"=w3884:errorcluster)  [unwired: 10 in]
                    n2289 = local write "TEMP RISE LAB01-1"(w3879) -> ()
                    n2290 = local write "FAIL LAB01-1"(w3882) -> ()
                    n2291 = local write "DISP LAB01-1"(w3878) -> ()
                    n2292 = local write "RESULT LAB01-1"(w3881) -> ()
                    n2293 = local write "data file error"(w3884) -> ()
                  }
                }
              }
              frame #1 {
                # "LAB01-2"
                n2294 = case shown="True" w3894 {
                  tunnel: w3896 -> [_ w3909]
                  tunnel: w3893 -> [_ w3906]
                  tunnel: w3895 -> [_ w3905]
                  frame False {
                  }
                  frame True {
                    n2295 = local read "TEMP START LAB01-2"() -> (w3911:cluster{"TL":dbl, "TN":dbl})
                    n2296 = local read "FAIL LAB01-2"() -> (w3902:cluster{"LO":dbl, "HI":dbl})
                    n2297 = local read "TDMS LAB01-2"() -> (w3910:refnum<k34>)
                    n2298 = local read "SET LAB01-2"() -> (w3907:T5)
                    n2299 = local read "DISP LAB01-2"() -> (w3908:T4)
                    n2300 = local read "RESULT LAB01-2"() -> (w3899:bool)
                    n2301 = local read "SIG LAB01-2"() -> (w3912:T2)
                    n2302 = Bundle("FAIL LAB01-2"=w3902, "SIG LAB01-2"=w3912, "TEMP START LAB01-2"=w3911, "DISP LAB01-2"=w3908, "SET LAB01-2"=w3907, "TDMS LAB01-2"=w3910) -> (w3897:T29)  [unwired: 1 in]
                    n2303 = call "sub vi - cycle&temp fail v6.vi"("Amps Lo?"=w3909, "Input Cluster"=w3897, "SELECT"=w3906, "Amps Hi?"=w3905, "Result In"=w3899) -> ("(FAIL) out"=w3901:cluster{"FAIL LO":dbl, "FAIL HI":dbl}, "(DISP) out"=w3904:T4, "T-RISE"=w3898:cluster{"T-RISE (L)":dbl, "T-RISE (N)":dbl}, "Result Out"=w3900:bool, "file error"=w3903:errorcluster)  [unwired: 10 in]
                    n2304 = local write "TEMP RISE LAB01-2"(w3898) -> ()
                    n2305 = local write "FAIL LAB01-2"(w3901) -> ()
                    n2306 = local write "DISP LAB01-2"(w3904) -> ()
                    n2307 = local write "RESULT LAB01-2"(w3900) -> ()
                    n2308 = local write "data file error"(w3903) -> ()
                  }
                }
              }
              frame #2 {
                # "LAB02-1"
                n2309 = case shown="True" w3914 {
                  tunnel: w3916 -> [_ w3929]
                  tunnel: w3913 -> [_ w3926]
                  tunnel: w3915 -> [_ w3925]
                  frame False {
                  }
                  frame True {
                    n2310 = local read "TEMP START LAB02-1"() -> (w3931:cluster{"TL":dbl, "TN":dbl})
                    n2311 = local read "FAIL LAB02-1"() -> (w3922:cluster{"LO":dbl, "HI":dbl})
                    n2312 = local read "TDMS LAB02-1"() -> (w3930:refnum<k34>)
                    n2313 = local read "SET LAB02-1"() -> (w3927:T5)
                    n2314 = local read "DISP LAB02-1"() -> (w3928:T4)
                    n2315 = local read "SIG LAB02-1"() -> (w3932:T2)
                    n2316 = local read "RESULT LAB02-1"() -> (w3919:bool)
                    n2317 = Bundle("FAIL LAB02-1"=w3922, "SIG LAB02-1"=w3932, "TEMP START LAB02-1"=w3931, "DISP LAB02-1"=w3928, "SET LAB02-1"=w3927, "TDMS LAB02-1"=w3930) -> (w3917:T30)  [unwired: 1 in]
                    n2318 = call "sub vi - cycle&temp fail v6.vi"("Amps Lo?"=w3929, "Input Cluster"=w3917, "SELECT"=w3926, "Amps Hi?"=w3925, "Result In"=w3919) -> ("(FAIL) out"=w3921:cluster{"FAIL LO":dbl, "FAIL HI":dbl}, "(DISP) out"=w3924:T4, "T-RISE"=w3918:cluster{"T-RISE (L)":dbl, "T-RISE (N)":dbl}, "Result Out"=w3920:bool, "file error"=w3923:errorcluster)  [unwired: 10 in]
                    n2319 = local write "TEMP RISE LAB02-1"(w3918) -> ()
                    n2320 = local write "FAIL LAB02-1"(w3921) -> ()
                    n2321 = local write "DISP LAB02-1"(w3924) -> ()
                    n2322 = local write "RESULT LAB02-1"(w3920) -> ()
                    n2323 = local write "data file error"(w3923) -> ()
                  }
                }
              }
              frame #3 {
                # "LAB02-2"
                n2324 = case shown="True" w3934 {
                  tunnel: w3936 -> [_ w3949]
                  tunnel: w3933 -> [_ w3946]
                  tunnel: w3935 -> [_ w3945]
                  frame False {
                  }
                  frame True {
                    n2325 = local read "TEMP START LAB02-2"() -> (w3951:cluster{"TL":dbl, "TN":dbl})
                    n2326 = local read "FAIL LAB02-2"() -> (w3942:cluster{"LO":dbl, "HI":dbl})
                    n2327 = local read "TDMS LAB02-2"() -> (w3950:refnum<k34>)
                    n2328 = local read "SET LAB02-2"() -> (w3947:T5)
                    n2329 = local read "DISP LAB02-2"() -> (w3948:T4)
                    n2330 = local read "SIG LAB02-2"() -> (w3952:T2)
                    n2331 = local read "RESULT LAB02-2"() -> (w3939:bool)
                    n2332 = Bundle("FAIL LAB02-2"=w3942, "SIG LAB02-2"=w3952, "TEMP START LAB02-2"=w3951, "DISP LAB02-2"=w3948, "SET LAB02-2"=w3947, "TDMS LAB02-2"=w3950) -> (w3937:T31)  [unwired: 1 in]
                    n2333 = call "sub vi - cycle&temp fail v6.vi"("Amps Lo?"=w3949, "Input Cluster"=w3937, "SELECT"=w3946, "Amps Hi?"=w3945, "Result In"=w3939) -> ("(FAIL) out"=w3941:cluster{"FAIL LO":dbl, "FAIL HI":dbl}, "(DISP) out"=w3944:T4, "T-RISE"=w3938:cluster{"T-RISE (L)":dbl, "T-RISE (N)":dbl}, "Result Out"=w3940:bool, "file error"=w3943:errorcluster)  [unwired: 10 in]
                    n2334 = local write "TEMP RISE LAB02-2"(w3938) -> ()
                    n2335 = local write "FAIL LAB02-2"(w3941) -> ()
                    n2336 = local write "DISP LAB02-2"(w3944) -> ()
                    n2337 = local write "RESULT LAB02-2"(w3940) -> ()
                    n2338 = local write "data file error"(w3943) -> ()
                  }
                }
              }
              frame #4 {
                # "LAB03-1"
                n2339 = case shown="True" w3954 {
                  tunnel: w3956 -> [_ w3969]
                  tunnel: w3953 -> [_ w3966]
